vi "Draw Horizontal Line 1D.vi"(4 "Alpha":dbl, 6 "Colour":u32(colorbox), 7 "Method":T1, 8 "Enable Alpha Blending (F)":bool, 9 "Point 2":T2, 10 "Point 1":T2, 11 "Pixel Data in":u32[](array[numeric])) -> (3 "Pixel Data out":u32[](array[numeric]))   [LabVIEW 2020, in "Raster (FPGA).lvlib"]
uses:
  Raster (FPGA).lvlib
  Libraries/Raster/Global 1.vi
  Libraries/3D/3D.lvlib
  Method.ctl
  Point 2D (I32).ctl
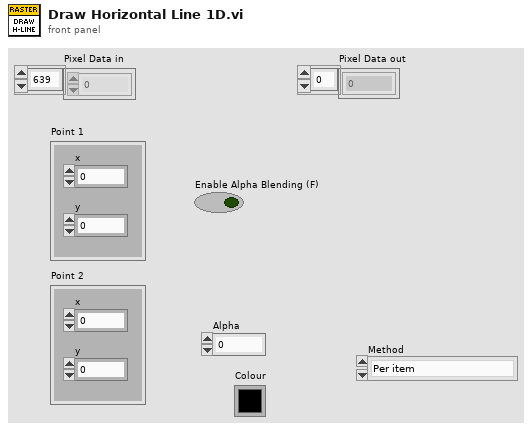
[diagram p1: front panel]
types:
  T1 = typedef "Raster (FPGA).lvlib/Method.ctl" = enum16{"Per item", "Row", "Replace Array Subset", "MoveBlock", " MoveBlock2 "}
  T2 = typedef "Raster (FPGA).lvlib/Point 2D (I32).ctl" = cluster{"x":i32, "y":i32}
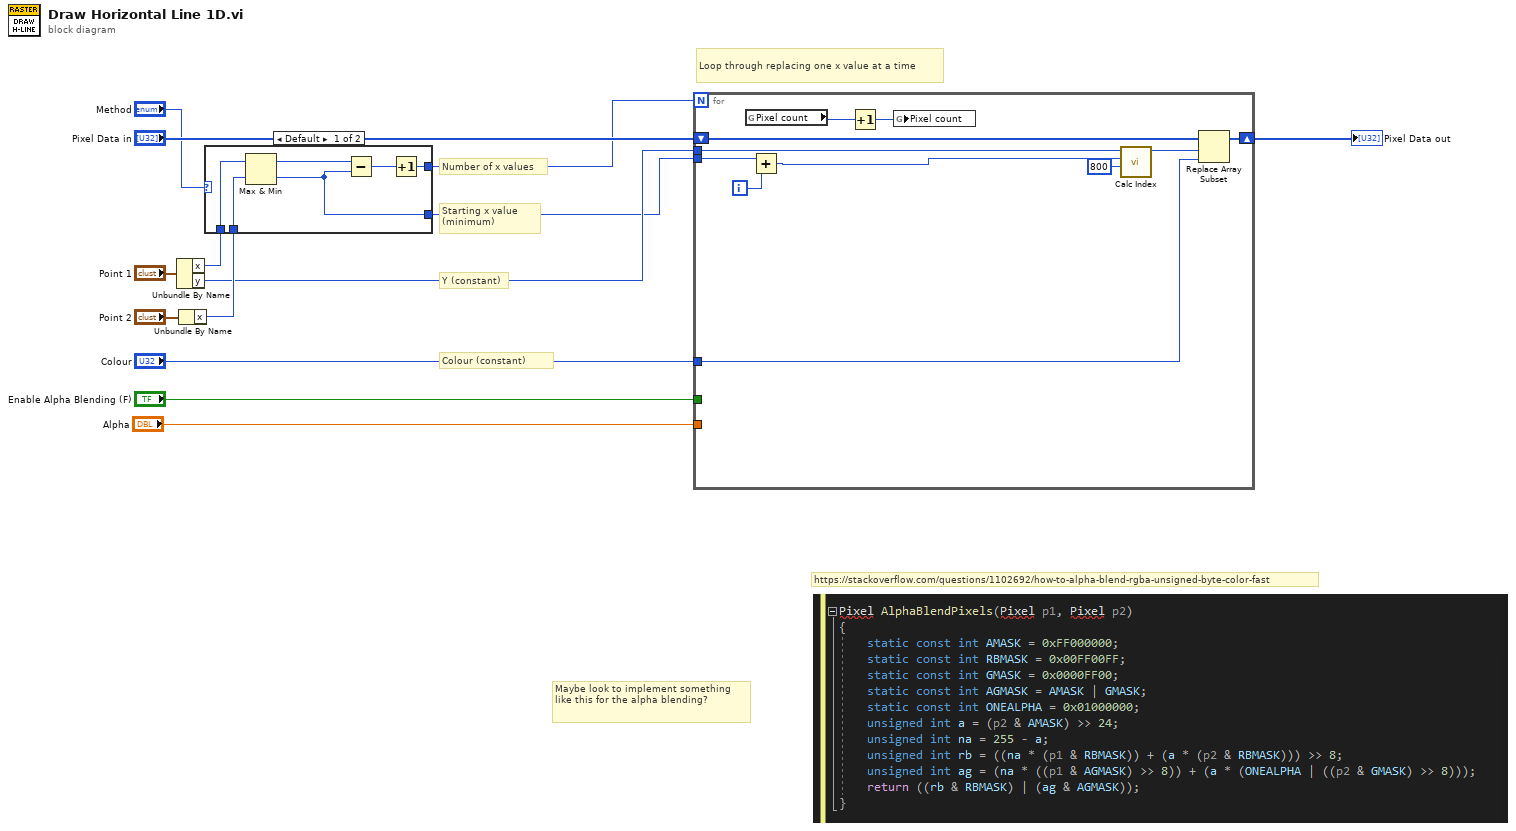
[diagram p0: block diagram]
diagram:
  # "Loop through replacing one x value at a time"
  # "Maybe look to implement something like this for the alpha blending?"
  # "https://stackoverflow.com/questions/1102692/how-to-alpha-blend-rgba-unsigned-byte-color-fast"
  # "Starting x value\n(minimum)"
  # "Number of x values"
  # "Colour (constant)"
  # "Y (constant)"
  n1 = Unbundle By Name("Point 1") -> ("x"=w4:i32, "y"=w8:i32)
  n2 = Unbundle By Name("Point 2") -> ("x"=w11:i32)
  n3 = case shown="Default" "Method" {
    tunnel: w11 -> [w18 w20]
    tunnel: [w16 w21] -> w9
    tunnel: [w15 w20] -> w7
    tunnel: w4 -> [w14 w21]
    frame Default {
      n4 = Max & Min(x=w14, y=w18) -> (max(x,y)=w17:i32, min(x,y)=w15:i32)
      n5 = Subtract(x=w17, y=w15) -> (x-y=w19:i32)
      n6 = Increment(x=w19) -> (x+1=w16:i32)
    }
    frame " MoveBlock2 " {
    }
  }
  n7 = for {
    N: w9 -> [_]
    tunnel: w7 -> [w31]
    tunnel: w8 -> [w25]
    shift-right: [w32] -> w5
    shift-left: "Pixel Data in" -> [w29]
    tunnel: "Colour" -> [w26]
    tunnel: "Enable Alpha Blending (F)" -> [_]
    tunnel: "Alpha" -> [_]
    i -> [w30]
    n8 = global read "Global 1.vi" "Pixel count"() -> (w28:u32)
    n9 = Add(x=w31, y=w30) -> (x+y=w24:i32)
    n10 = Increment(x=w28) -> (x+1=w27:u32)
    n11 = global write "Global 1.vi" "Pixel count"(w27) -> ()
    n12 = call "Calc Index.vi"("Cols Per Row"=800, "Col"=w24, "Row"=w25) -> ("Index"=w23:i32)  [unwired: 8 in]
    n13 = Replace Array Subset(array=w29, new element=w26, index=w23) -> (w32:u32[])
  }
  "Pixel Data out" <- w5
